vi "AIT 664 - Add Multiple Channels.vi"(8 "error in (no error)":errorcluster, 11 "Node Ptr":u64 format="%.0x") -> (0 "error out":errorcluster)   [LabVIEW 2013, in "AIT 664 Custom Device.lvlib"]
uses:
  AIT 664 Custom Device.lvlib
  Controls/Channel Setup.ctl
  <vilib>/NI Veristand/Custom Device API/Custom Device Channel Type.ctl
  <vilib>/NI Veristand/Custom Device API/Custom Device Channel.ctl
  Controls and Global/Global.vi
  <vilib>/NI Veristand/Custom Device API/Get Item Property (U32 Array).vi
  <vilib>/NI Veristand/Custom Device API/Get Item Property (Boolean).vi
  <vilib>/NI Veristand/Custom Device API/Custom Device API.lvlib
panel:
  in  "Cancel":bool
  in  "OK":bool
  in  "Parameters to Add":T1[](array[typedef]) {"Scale Offset" format="%.2f"; "Scale Factor" format="%.2f"; "Number of Bits" min=1 max=32 step=1; "Start Bit" min=0 max=31 step=1; "First Byte" min=1 max=31 step=1}
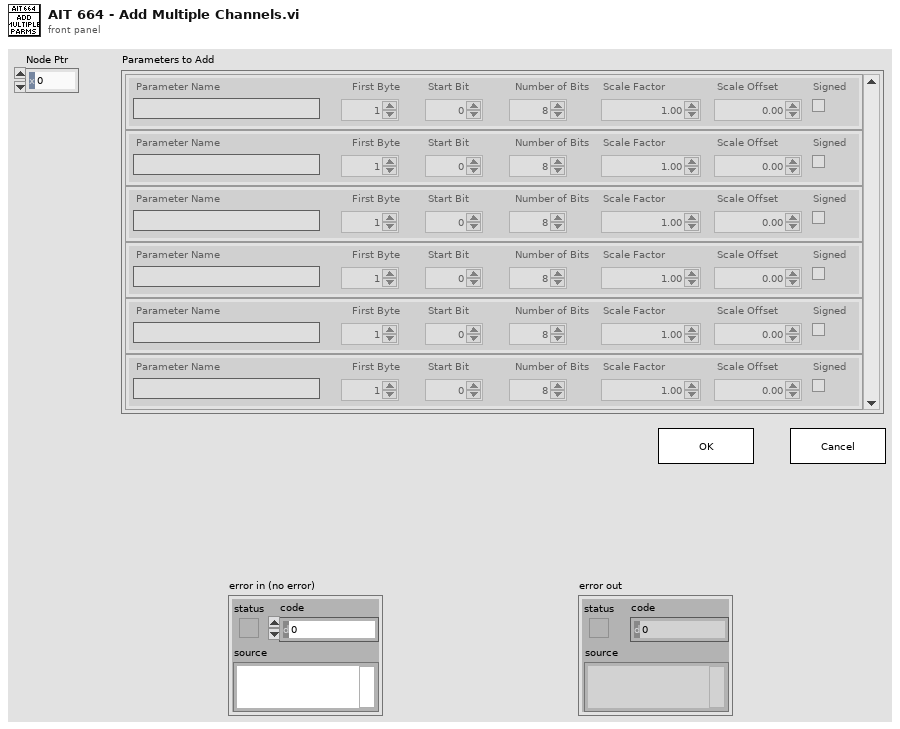
[diagram p1: front panel]
types:
  T1 = typedef "AIT 664 Custom Device.lvlib/Channel Setup.ctl" = cluster{"Parameter Name":string, "First Byte":i32, "Start Bit":i32, "Number of Bits":i32, "Scale Factor":dbl, "Scale Offset":dbl, "Signed":bool}
  T2 = typedef "Custom Device API.lvlib/Custom Device Channel Type.ctl" = enum16{"Input", "Output"}
  T3 = typedef "Custom Device API.lvlib/Custom Device Channel.ctl" = cluster{"Type":T2, "Units":string, "Default Value":dbl, "Faultable":bool, "Scalable":bool}
  T4 = typedef "Custom Device API.lvlib/Custom Device Item Ref.ctl" = u64
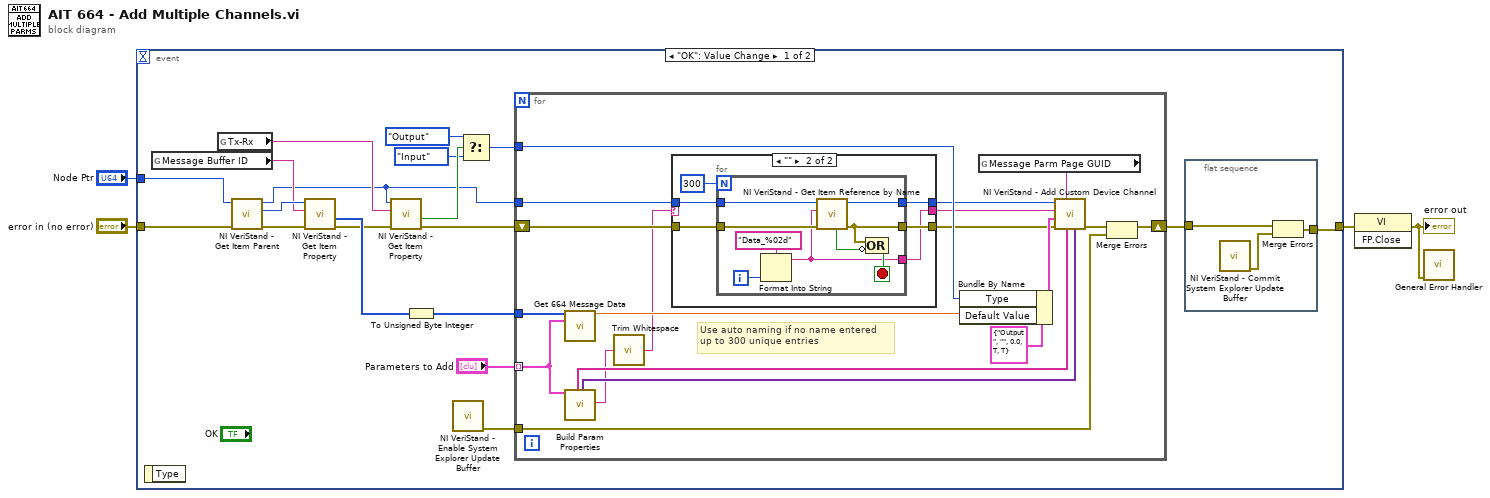
[diagram p0: block diagram]
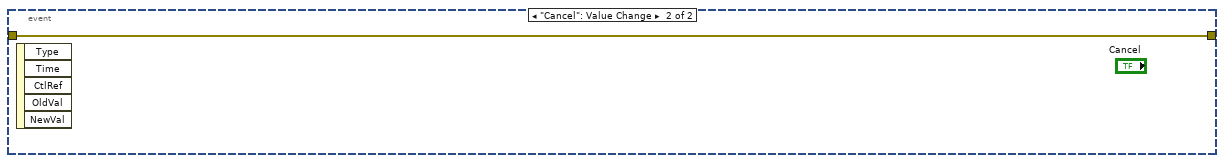
[diagram p3: hidden frame]
diagram:
  n1 = event shown="[0] \"OK\": Value Change" {
    selector: _ -> [_ _]
    dyn-events: _ -> [_ _]
    timeout: _ -> [_ _]
    tunnel: [w23 w64] -> w2
    tunnel: "error in (no error)" -> [w9 w64]
    tunnel: "Node Ptr" -> [w10 _]
    event "OK": Value Change {
      n2 = event-data() -> ()  [unwired: 1 in, 1 out]
      n3 = global read "Global.vi" "Message Buffer ID"() -> (w20:string)
      n4 = global read "Global.vi" "Tx-Rx"() -> (w16:string)
      n5 = call <vilib>:"NI VeriStand - Get Item Parent.vi"("error in (no error)"=w9, "Item Ref in"=w10) -> ("error out"=w21:errorcluster, "Parent Ref"=w22:T4, "Item Ref out"=w5:T4)  [unwired: 6 in, 1 out]
      n6 = call-poly <vilib>:"NI VeriStand - Get Item Property.vi"("error in (no error)"=w21, "Property Name"=w20, "Item Ref in"=w22) -> ("error out"=w17:errorcluster, "Value"=w19:u32[])  [unwired: 5 in, 2 out]
      n7 = call-poly <vilib>:"NI VeriStand - Get Item Property.vi"("error in (no error)"=w17, "Property Name"=w16, "Item Ref in"=w5) -> ("error out"=w11:errorcluster, "Value"=w15:bool)  [unwired: 5 in, 2 out]
      n8 = To Unsigned Byte Integer(number=w19) -> (unsigned 8bit integer=w18:u8[])
      n9 = call <vilib>:"NI VeriStand - Enable System Explorer Update Buffer.vi"() -> ("error out"=w8:errorcluster)  [unwired: 11 in]
      n10 = Select(t=Custom_Device_Channel_Type."Output" ("Type"), s=w15, f=Custom_Device_Channel_Type."Input" ("Type")) -> (s? t:f=w12:T2)
      n11 = for {
        tunnel: w18 -> [w39]
        tunnel: w12 -> [w36]
        tunnel: w5 -> [w31]
        tunnel: w8 -> [w25]
        tunnel: "Parameters to Add" -> [w30] mode=indexing
        shift-right: [w24] -> w6
        shift-left: w11 -> [w34]
        # "Use auto naming if no name entered\nup to 300 unique entries"
        n12 = call "Get 664 Message Data.vi"("MSG DATA"=w39, "664 Parameter"=w30) -> ("Value"=w38:dbl)  [unwired: 12 in, 1 out]
        n13 = call "Build Param Properties.vi"("Parameter"=w30) -> ("Prop Names"=w41:string[], "Prop Values"=w40:variant[], "name"=w29:string)  [unwired: 10 in, 6 out]
        n14 = call <vilib>:"Trim Whitespace.vi"("string"=w29) -> ("trimmed string"=w27:string)  [unwired: 1 in]
        n15 = case shown="\"\"" w27 {
          selector: w27 -> [w45 _]
          tunnel: w34 -> [w43 w51]
          tunnel: [w43 w50] -> w33
          tunnel: [w44 w49] -> w32
          tunnel: w31 -> [w44 w47]
          tunnel: [w45 w46] -> w28
          frame Default {
            # "Valid Name String Entered"
          }
          frame "" {
            n16 = for {
              N: 300 -> [_]
              tunnel: w47 -> [w60]
              tunnel: w51 -> [w59]
              tunnel: [w57] -> w50
              tunnel: [w55] -> w49
              tunnel: [w52] -> w46
              i -> [w54]
              stop <- w58 stop-if-true
              n17 = Format Into String(format string="Data_%02d" ("name"), w54) -> (resulting string=w52:string)  [unwired: 2 in, 1 out]
              n18 = call <vilib>:"NI VeriStand - Get Item Reference by Name.vi"("error in (no error)"=w59, "Item Name"=w52, "Parent Ref in"=w60) -> ("error out"=w57:errorcluster, "Parent Ref out"=w55:T4, "Found"=w56:bool)  [unwired: 5 in, 1 out]
              n19 = Compound Arithmetic op=OR(w57, invert w56) -> (w58:bool)
            }
          }
        }
        n20 = Bundle By Name(cluster=T3 {"Type"=enum."Output", "Units"="", "Default Value"=0.0, "Faultable"=TRUE, "Scalable"=TRUE} ("Channel"), "Type"=w36, "Default Value"=w38) -> (w35:T3)
        n21 = global read "Global.vi" "Message Parm Page GUID"() -> (w42:string)
        n22 = call <vilib>:"NI VeriStand - Add Custom Device Channel.vi"("Property Values"=w40, "Property names"=w41, "GUID (Default Channel)"=w42, "error in (no error)"=w33, "Channel"=w35, "Channel Name"=w28, "Parent Ref in"=w32) -> ("error out"=w26:errorcluster)  [unwired: 1 in, 3 out]
        n23 = Merge Errors(w26, w25) -> (w24:errorcluster)
      }
      n24 = flat-sequence {
        tunnel: w6 -> [w63]
        tunnel: [w61] -> w23
        frame #0 {
          n25 = call <vilib>:"NI VeriStand - Commit System Explorer Update Buffer.vi"() -> ("error out"=w62:errorcluster)  [unwired: 11 in]
          n26 = Merge Errors(w63, w62) -> (w61:errorcluster)
        }
      }
    }
    event "Cancel": Value Change {
      n27 = event-data() -> ()  [unwired: 1 in, 5 out]
    }
  }
  n28 = invoke class="VI" method="FP.Close"(error in=w2) -> (error out=w1:errorcluster)  [unwired: 2 in, 2 out]
  "error out" <- w1
  n29 = call <vilib>:"General Error Handler.vi"("error in (no error)"=w1) -> ()  [unwired: 10 in, 5 out]
